vi "Read Car Wash Controller.vi"(8 "error in (no error)":errorcluster, 11 "Entry Console in":refnum<class "Entry Console.lvclass">) -> (0 "error out":errorcluster, 2 "Architecture.lvlib:Queue.lvclass":refnum<class "Queue.lvclass">, 3 "Entry Console out":refnum<class "Entry Console.lvclass">)   [LabVIEW 2012, in "Entry Console.lvlib" / "Entry Console.lvclass"]
uses:
  Entry Console.lvclass
  Queue/Queue.lvclass
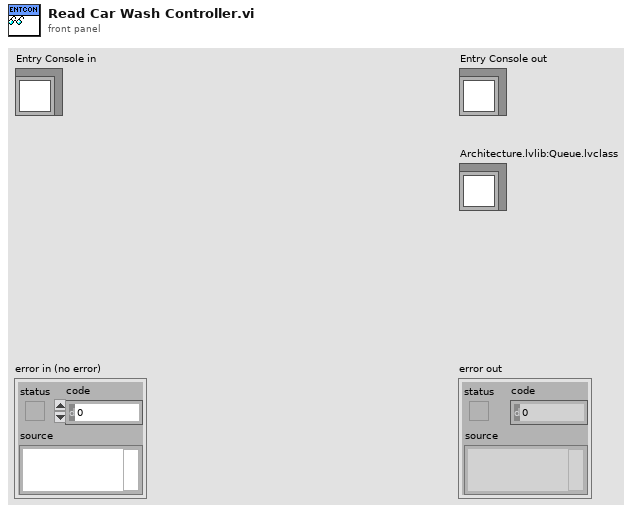
[diagram p1: front panel]
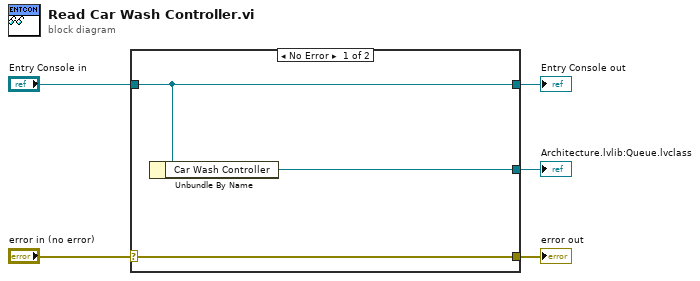
[diagram p0: block diagram]
diagram:
  n1 = case shown="No Error" "error in (no error)" {
    selector: "error in (no error)" -> [w8 w9]
    tunnel: [w8 w9] -> w4
    tunnel: [w7 w10] -> w2
    tunnel: "Entry Console in" -> [w7 w10]
    tunnel: [w6 _] -> w1
    frame No Error {
      n2 = Unbundle By Name(w7) -> ("Car Wash Controller"=w6:refnum<class "Queue.lvclass">)
    }
    frame Error {
    }
  }
  "error out" <- w4
  "Entry Console out" <- w2
  "Architecture.lvlib:Queue.lvclass" <- w1
